vi "client.vi"() -> ()   [LabVIEW 2020]
panel:
  in  "stop":bool
  in  "Tamper":bool
  in  "Alarm":bool
  in  "Bypass":bool
  # "Zone 1"
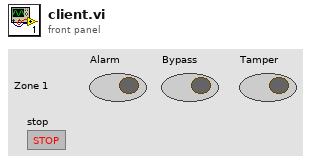
[diagram p1: front panel]
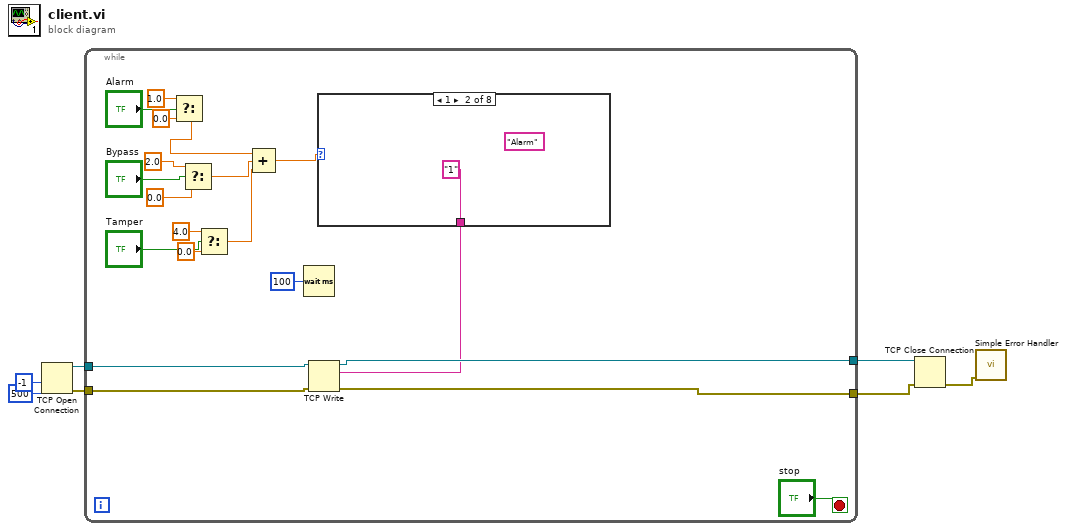
[diagram p0: block diagram]
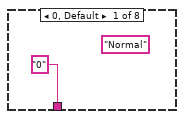
[diagram p2: hidden frame]
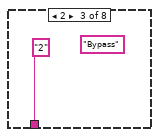
[diagram p3: hidden frame]
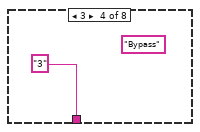
[diagram p4: hidden frame]
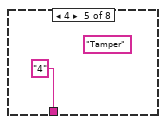
[diagram p5: hidden frame]
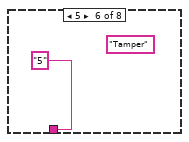
[diagram p6: hidden frame]
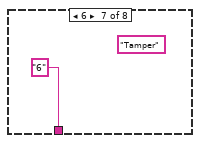
[diagram p7: hidden frame]
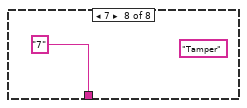
[diagram p8: hidden frame]
diagram:
  n1 = TCP Open Connection(remote port or service name=u16 500, timeout ms (60000)=-1) -> (connection ID=w7:refnum<k5>, error out=w6:errorcluster)  [unwired: 3 in]
  n2 = while {
    tunnel: w7 -> [w13]
    tunnel: w6 -> [w12]
    tunnel: [w11] -> w5
    tunnel: [w10] -> w4
    stop <- "stop" stop-if-true
    n3 = Select(t=1.0, s="Alarm", f=0.0) -> (s? t:f=w27:dbl)
    n4 = Select(t=2.0, s="Bypass", f=0.0) -> (s? t:f=w20:dbl)
    n5 = Select(t=4.0, s="Tamper", f=0.0) -> (s? t:f=w16:dbl)
    n6 = Compound Arithmetic op=ADD(w27, w20, w16) -> (w15:dbl)
    n7 = Wait (ms)(milliseconds to wait=u32 100) -> ()  [unwired: 1 out]
    n8 = case shown="1" w15 {
      tunnel: ["0" "1" "2" "3" "4" "5" "6" "7"] -> w9
      frame 0, Default {
        (unwired) "Normal"
      }
      frame 1 {
        (unwired) "Alarm"
      }
      frame 2 {
        (unwired) "Bypass"
      }
      frame 3 {
        (unwired) "Bypass"
      }
      frame 4 {
        (unwired) "Tamper"
      }
      frame 5 {
        (unwired) "Tamper"
      }
      frame 6 {
        (unwired) "Tamper"
      }
      frame 7 {
        (unwired) "Tamper"
      }
    }
    n9 = TCP Write(connection ID=w13, data in=w9, error in (no error)=w12) -> (connection ID out=w11:refnum<k5>, error out=w10:errorcluster)  [unwired: 1 in, 1 out]
  }
  n10 = TCP Close Connection(connection ID=w5, error in (no error)=w4) -> (error out=w1:errorcluster)  [unwired: 1 in, 1 out]
  n11 = call <vilib>:"Simple Error Handler.vi"("error in (no error)"=w1) -> ()  [unwired: 4 in, 5 out]
